vi "Status Log FGV.vi"(7 "Action":T1=enum."Show Status File", 8 "error in":errorcluster, 10 "Status":string) -> (0 "error out":errorcluster)   [LabVIEW 2014]
uses:
  Status Log.ctl
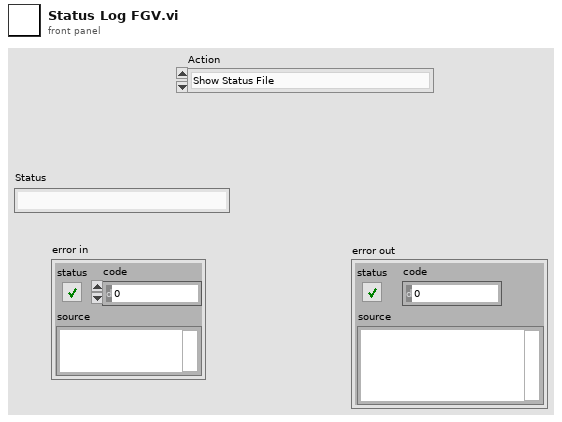
[diagram p1: front panel]
types:
  T1 = typedef "Status Log.ctl" = enum16{"Close file", "Open Status file", "Add Status", "Show Status File"}
  T2 = enum16{"open", "replace", "create", "open or create", "replace or create", "replace or create with confirmation"}
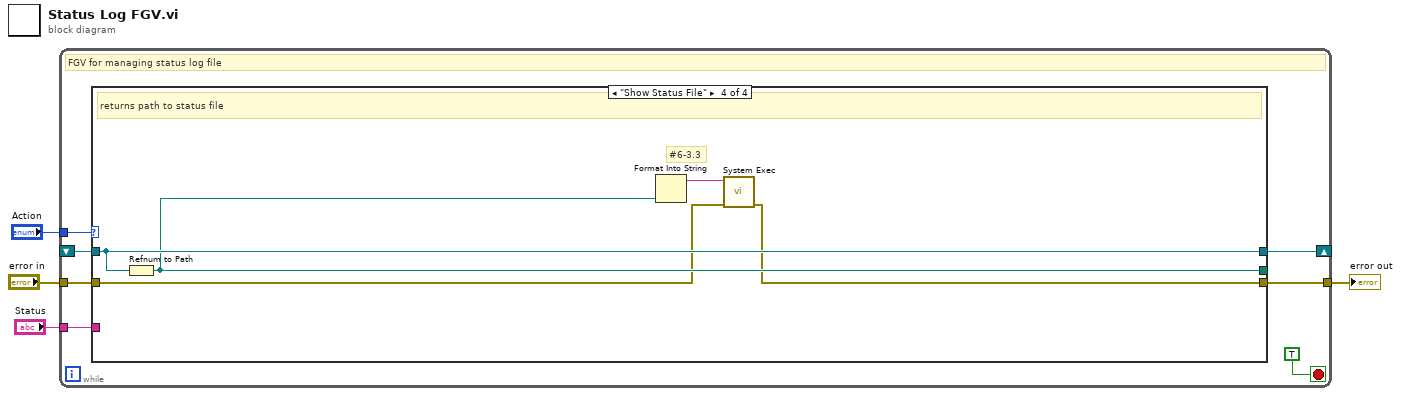
[diagram p0: block diagram]
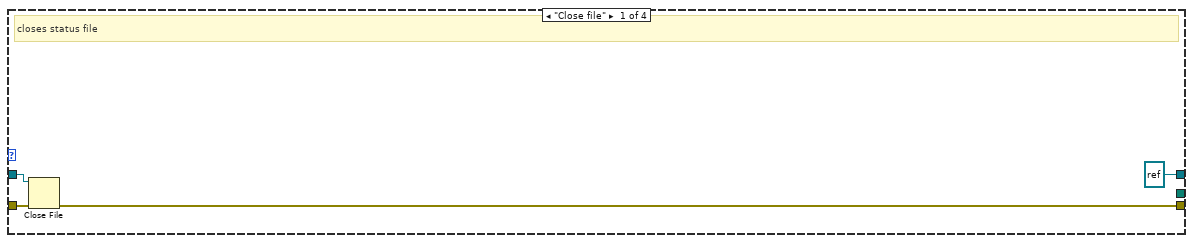
[diagram p2: hidden frame]
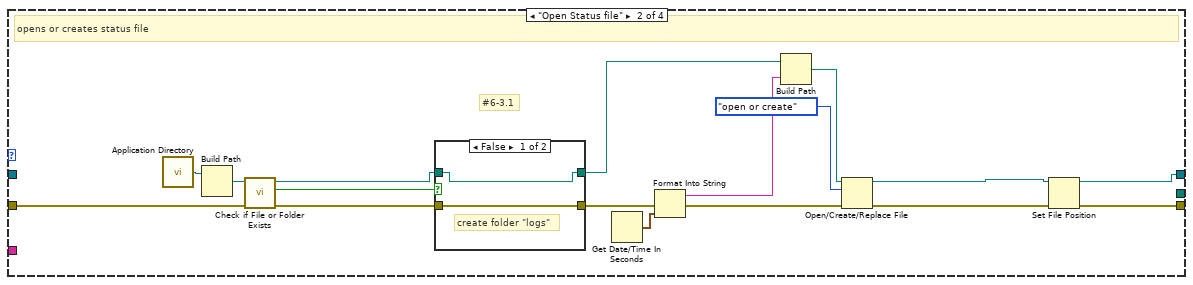
[diagram p3: hidden frame]
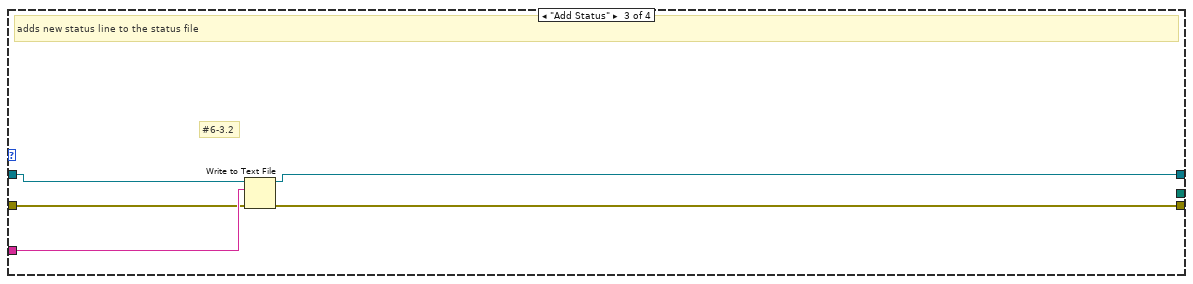
[diagram p5: hidden frame]
diagram:
  n1 = while {
    tunnel: "Action" -> [w10]
    tunnel: "Status" -> [w9]
    tunnel: [w8] -> w2
    tunnel: "error in" -> [w7]
    shift-right: [w5] -> _
    shift-left: _ -> [w6]
    stop <- TRUE stop-if-true
    # "FGV for managing status log file"
    n2 = case shown="\"Show Status File\"" w10 {
      tunnel: w9 -> [_ _ w38 _]
      tunnel: [w14 w24 w41 w42] -> w8
      tunnel: w7 -> [w15 w17 w37 w43]
      tunnel: [refnum<file> refnum ("refnum out") w23 w40 w46] -> w5
      tunnel: w6 -> [w13 _ w39 w46]
      tunnel: [_ _ _ w44] -> _
      frame "Close file" {
        # "closes status file"
        n3 = Close File(refnum=w13, error in=w15) -> (error out=w14:errorcluster)  [unwired: 1 out]
      }
      frame "Open Status file" {
        # "#6-3.1"
        # "opens or creates status file"
        n4 = call <vilib>:"Application Directory.vi"() -> ("Application Directory"=w32:path)
        n5 = Build Path(base path=w32) -> (appended path=w22:path)  [unwired: 1 in]
        n6 = call <vilib>:"Check if File or Folder Exists.vi"("error in (no error)"=w17, "path"=w22) -> ("error out"=w18:errorcluster, "file or folder exists?"=w21:bool, "dup path"=w20:path)  [unwired: 7 in]
        n7 = case shown="False" w21 {
          tunnel: w20 -> [w34 w36]
          tunnel: [w34 w36] -> w19
          tunnel: w18 -> [w33 w35]
          tunnel: [w33 w35] -> w16
          frame False {
            # "create folder \"logs\""
          }
          frame True {
          }
        }
        n8 = Get Date/Time In Seconds() -> (seconds since 1Jan1904=w31:timestamp)
        n9 = Format Into String "Format Into String"(error in=w16, w31) -> (resulting string=w29:string, error out=w30:errorcluster)  [unwired: 2 in]
        n10 = Build Path(base path=w19, name or relative path=w29) -> (appended path=w28:path)
        n11 = Open/Create/Replace File(file path (use dialog)=w28, error in=w30, operation (0:open)=T2."open or create") -> (refnum out=w25:refnum<file>, error out=w26:errorcluster)  [unwired: 3 in, 1 out]
        n12 = Set File Position(refnum=w25, error in=w26) -> (refnum out=w23:refnum<file>, error out=w24:errorcluster)  [unwired: 2 in]
      }
      frame "Add Status" {
        # "#6-3.2"
        # "adds new status line to the status file"
        n13 = Write to Text File(file (use dialog)=w39, text=w38, error in=w37) -> (refnum out=w40:refnum<file>, error out=w41:errorcluster)  [unwired: 1 in, 1 out]
      }
      frame "Show Status File" {
        # "#6-3.3"
        # "returns path to status file"
        n14 = Refnum to Path(1:w46) -> (0:w44:path)
        n15 = Format Into String(w44) -> (resulting string=w45:string)  [unwired: 3 in, 1 out]
        n16 = call <vilib>:"System Exec.vi"("error in (no error)"=w43, "command line"=w45) -> ("error out"=w42:errorcluster)  [unwired: 6 in, 3 out]
      }
    }
  }
  "error out" <- w2
